vi "SDT_WriteFile.vi"(5 "ActiveModule":string[](array[string]), 7 "Data":T12, 8 "ErrorIn":errorcluster, 9 "SPCdata":T13={"base_adr"=52672, "init"=0, "cfd_limit_low"=-0.0, "cfd_limit_high"=5.019608, "cfd_zc_level"=-5.2913384, "cfd_holdoff"=5.0, "sync_zc_level"=-5.2913384, "sync_holdoff"=4.0, "sync_threshold"=-70.588234, "tac_range"=50.033573, "sync_freq_div"=1, "tac_gain"=1, "tac_offset"=5.098039, "tac_limit_low"=0.0, "tac_limit_high"=100.0, "adc_resolution"=12, "ext_latch_delay"=0, "collect_time"=1.0, "display_time"=1.0, "repeat_time"=10.0, "stop_on_time"=1, "stop_on_ovfl"=1, "dither_range"=128, "count_incr"=1, "mem_bank"=0, "dead_time_comp"=0, "scan_control"=0, "routing_mode"=0, "tac_enable_hold"=0.0, "pci_card_no"=-1, "mode"=5, "scan_size_x"=1, "scan_size_y"=1, "scan_rout_x"=1, "scan_rout_y"=1, "scan_flyback"=65537, "scan_borders"=0, "scan_polarity"=0, "pixel_clock"=1, "line_compression"=1, "trigger"=0, "pixel_time"=1e-07, "ext_pixclk_div"=1, "rate_count_time"=1.0, "macro_time_clk"=0, "add_select"=0, "test_eep"=1, "adc_zoom"=0, "img_size_x"=1, "img_size_y"=1, "img_rout_x"=1, "img_rout_y"=1, "xy_gain"=1, "master_clock"=0, "adc_sample_delay"=0, "detector_type"=1, "chan_enable"=4191231, "chan_slope"=0, "chan_spec_no"=34835, "tdc_control"=0, "tdc_offset1"=0.0, "tdc_offset2"=0.0, "tdc_offset3"=0.0, "tdc_offset4"=0.0, "tdc_offset5"=0.0, "tdc_offset6"=0.0, "cfd_th5_tdc"=0.0, "cfd_th6_tdc"=0.0, "cfd_zc5_tdc"=0.0, "cfd_zc6_tdc"=0.0, "future_reserve1"=0, "future_reserve2"=0, "future_reserve3"=0, "future_reserve4"=0} {"scan_flyback" format="%x"}, 10 "ImageSize":i32=256, 11 "SDT-FilePath":path=path "\\\\lab13\\C/Users/jannis/Desktop/ZeissFifo.sdt") -> (0 "ErrorOut":errorcluster)   [LabVIEW 2017]
doc: "This VI writes a SDT-file to disc. The SetUp and the MeasureInfo blocks are created and appended with the data blocks. \nThis VI is limited to writing a DecayMatrix from a FIFO-Image recording and optional an IntensityImage to file. For single mode recordings use the spcmdll VI \\Public\\Configure\\Memory Transfer\\SPC_save_data_to_sdtfile.vi.\nFor a description of the format for the Data input cluster to this VI see the usage in \\Example\\ImagingEventStream-SimpleFifoImage.vi. Leave either of the cluster input arrays empty to not save them to disc.\nFor a description of the *.sdt file format see: SPC_data_file_structure.h\n\ninfo@becker-hickl.com"
uses:
  SPC_Wrappers/SPC_Controls/bhfile_header.ctl
  SPC_Wrappers/SPC_Controls/SPCdata.ctl
  SPC_Wrappers/SPC_Controls/MeasureInfo.ctl
  SPC_Wrappers/SPC_Controls/MeasureInfo_PartB.ctl
  SPC_Wrappers/SPC_Controls/MeasStopInfo.ctl
  SPC_Wrappers/SPC_Controls/MeasFCSInfo.ctl
  SPC_Wrappers/SPC_Controls/MeasureInfo_PartE.ctl
  SPC_Wrappers/SPC_Controls/MeasHISTInfo.ctl
  SPC_Wrappers/SPC_Controls/HISTInfoExt.ctl
  SPC_Wrappers/SPC_Controls/MeasureInfo_PartI.ctl
  SPC_Wrappers/SPC_Controls/MeasureInfo_PartK.ctl
  SPC_Wrappers/SPC_Controls/MeasureInfo_PartM.ctl
  SPC_Wrappers/SPC_Controls/BHFileBlockHeader.ctl
  SPC_Wrappers/SPC_Controls/FileType.ctl
  SDT_CreateModTypeString.vi
  SDT_MeasureBlockToString.vi
panel:
  out "Info Block":string
  out "BHFileBlockHeaders":T1[](array[typedef])
  out "MeasureInfos":T2[](array[typedef]) {"MeasStopInfo"."flags" format="x%x"}
  out "BlockLengths":i32[](array[numeric])
  out "bhfile_header":T14 {"chksum" format="x%x"; "header_valid" format="x%x"}
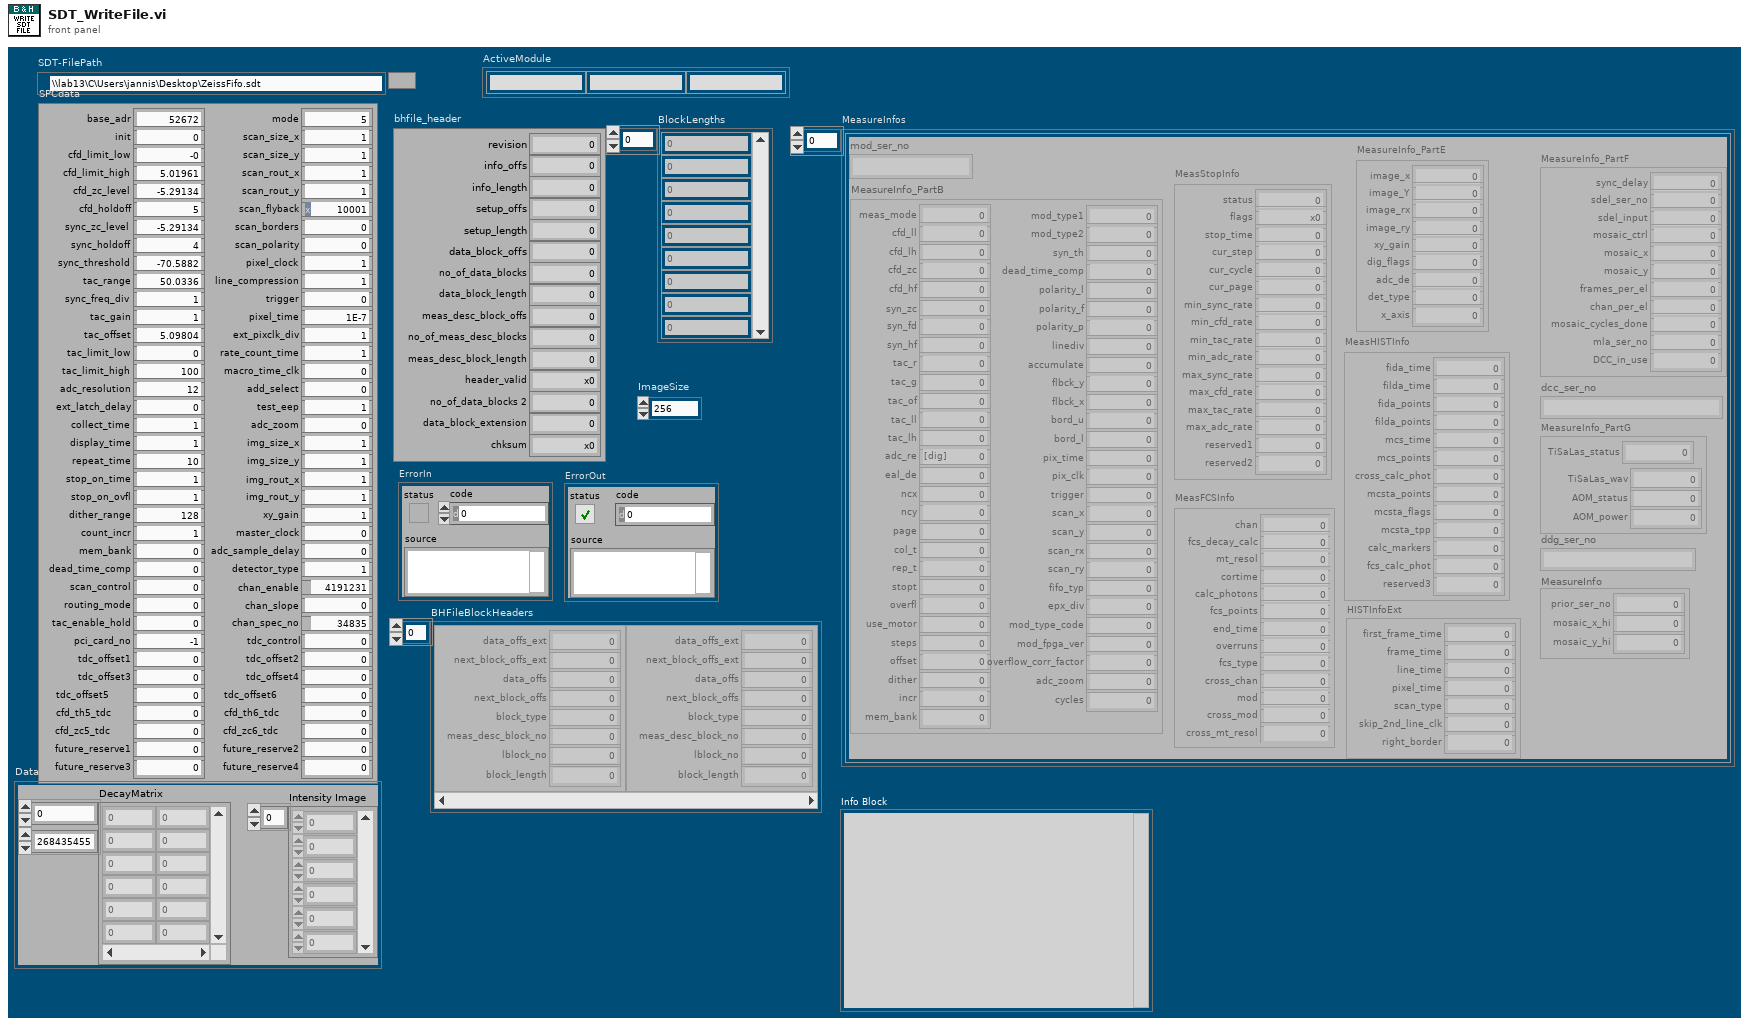
[diagram p1: front panel]
types:
  T1 = typedef "BHFileBlockHeader.ctl" = cluster{"data_offs_ext":u8, "next_block_offs_ext":u8, "data_offs":u32, "next_block_offs":u32, "block_type":u16, "meas_desc_block_no":i16, "lblock_no":u32, "block_length":u32}
  T2 = typedef "MeasureInfo.ctl" = cluster{"mod_ser_no":string, "MeasureInfo_PartB":T3, "MeasStopInfo":T4, "MeasFCSInfo":T5, "MeasureInfo_PartE":T6, "MeasHISTInfo":T7, "HISTInfoExt":T8, "MeasureInfo_PartF":T9, "dcc_ser_no":string, "MeasureInfo_PartG":T10, "ddg_ser_no":string, "MeasureInfo":T11}
  T3 = typedef "MeasureInfo_PartB.ctl" = cluster{"meas_mode":i16, "cfd_ll":sgl, "cfd_lh":sgl, "cfd_zc":sgl, "cfd_hf":sgl, "syn_zc":sgl, "syn_fd":i16, "syn_hf":sgl, "tac_r":sgl, "tac_g":i16, "tac_of":sgl, "tac_ll":sgl, "tac_lh":sgl, "adc_re":i16, "eal_de":i16, "ncx":i16, "ncy":i16, "page":u16, "col_t":sgl, "rep_t":sgl, "stopt":i16, "overfl":i8, "use_motor":i16, "steps":u16, "offset":sgl, "dither":i16, "incr":i16, "mem_bank":i16, "mod_type1":u64, "mod_type2":u64, "syn_th":sgl, "dead_time_comp":i16, "polarity_l":i16, "polarity_f":i16, "polarity_p":i16, "linediv":i16, "accumulate":i16, "flbck_y":i32, "flbck_x":i32, "bord_u":i32, "bord_l":i32, "pix_time":sgl, "pix_clk":i16, "trigger":i16, "scan_x":i32, "scan_y":i32, "scan_rx":i32, "scan_ry":i32, "fifo_typ":i16, "epx_div":i32, "mod_type_code":u16, "mod_fpga_ver":u16, "overflow_corr_factor":sgl, "adc_zoom":i32, "cycles":i32}
  T4 = typedef "MeasStopInfo.ctl" = cluster{"status":u16, "flags":u16, "stop_time":sgl, "cur_step":i32, "cur_cycle":i32, "cur_page":i32, "min_sync_rate":sgl, "min_cfd_rate":sgl, "min_tac_rate":sgl, "min_adc_rate":sgl, "max_sync_rate":sgl, "max_cfd_rate":sgl, "max_tac_rate":sgl, "max_adc_rate":sgl, "reserved1":i32, "reserved2":sgl}
  T5 = typedef "MeasFCSInfo.ctl" = cluster{"chan":u16, "fcs_decay_calc":u16, "mt_resol":u32, "cortime":sgl, "calc_photons":u32, "fcs_points":i32, "end_time":sgl, "overruns":u16, "fcs_type":u16, "cross_chan":u16, "mod":u16, "cross_mod":u16, "cross_mt_resol":u32}
  T6 = typedef "MeasureInfo_PartE.ctl" = cluster{"image_x":i32, "image_Y":i32, "image_rx":i32, "image_ry":i32, "xy_gain":i16, "dig_flags":i16, "adc_de":i16, "det_type":i16, "x_axis":i16}
  T7 = typedef "MeasHISTInfo.ctl" = cluster{"fida_time":sgl, "filda_time":sgl, "fida_points":i32, "filda_points":i32, "mcs_time":sgl, "mcs_points":i32, "cross_calc_phot":u32, "mcsta_points":u16, "mcsta_flags":u16, "mcsta_tpp":u32, "calc_markers":u32, "fcs_calc_phot":u32, "reserved3":u32}
  T8 = typedef "HISTInfoExt.ctl" = cluster{"first_frame_time":sgl, "frame_time":sgl, "line_time":sgl, "pixel_time":sgl, "scan_type":i16, "skip_2nd_line_clk":i16, "right_border":u32}
  T9 = typedef "MeasureInfo_PartI.ctl" = cluster{"sync_delay":sgl, "sdel_ser_no":u16, "sdel_input":i8, "mosaic_ctrl":i8, "mosaic_x":u8, "mosaic_y":u8, "frames_per_el":i16, "chan_per_el":i16, "mosaic_cycles_done":i32, "mla_ser_no":u16, "DCC_in_use":u8}
  T10 = typedef "MeasureInfo_PartK.ctl" = cluster{"TiSaLas_status":u16, "TiSaLas_wav":u16, "AOM_status":u8, "AOM_power":u8}
  T11 = typedef "MeasureInfo_PartM.ctl" = cluster{"prior_ser_no":i32, "mosaic_x_hi":u8, "mosaic_y_hi":u8}
  T12 = cluster{"DecayMatrix":u16[][], "Intensity Image":u32[]}
  T13 = typedef "SPCdata.ctl" = cluster{"base_adr":u16, "init":i16, "cfd_limit_low":sgl, "cfd_limit_high":sgl, "cfd_zc_level":sgl, "cfd_holdoff":sgl, "sync_zc_level":sgl, "sync_holdoff":sgl, "sync_threshold":sgl, "tac_range":sgl, "sync_freq_div":i16, "tac_gain":i16, "tac_offset":sgl, "tac_limit_low":sgl, "tac_limit_high":sgl, "adc_resolution":i16, "ext_latch_delay":i16, "collect_time":sgl, "display_time":sgl, "repeat_time":sgl, "stop_on_time":i16, "stop_on_ovfl":i16, "dither_range":i16, "count_incr":i16, "mem_bank":i16, "dead_time_comp":i16, "scan_control":u16, "routing_mode":u16, "tac_enable_hold":sgl, "pci_card_no":i16, "mode":u16, "scan_size_x":u32, "scan_size_y":u32, "scan_rout_x":u32, "scan_rout_y":u32, "scan_flyback":u32, "scan_borders":u32, "scan_polarity":u16, "pixel_clock":u16, "line_compression":u16, "trigger":u16, "pixel_time":sgl, "ext_pixclk_div":u32, "rate_count_time":sgl, "macro_time_clk":i16, "add_select":i16, "test_eep":i16, "adc_zoom":i16, "img_size_x":u32, "img_size_y":u32, "img_rout_x":u32, "img_rout_y":u32, "xy_gain":i16, "master_clock":i16, "adc_sample_delay":i16, "detector_type":i16, "chan_enable":u32, "chan_slope":u32, "chan_spec_no":u32, "tdc_control":u32, "tdc_offset1":sgl, "tdc_offset2":sgl, "tdc_offset3":sgl, "tdc_offset4":sgl, "tdc_offset5":sgl, "tdc_offset6":sgl, "cfd_th5_tdc":sgl, "cfd_th6_tdc":sgl, "cfd_zc5_tdc":sgl, "cfd_zc6_tdc":sgl, "future_reserve1":u64, "future_reserve2":u64, "future_reserve3":u64, "future_reserve4":u64}
  T14 = typedef "bhfile_header.ctl" = cluster{"revision":i16, "info_offs":i32, "info_length":i16, "setup_offs":i32, "setup_length":u16, "data_block_offs":i32, "no_of_data_blocks":i16, "data_block_length":u32, "meas_desc_block_offs":i32, "no_of_meas_desc_blocks":i16, "meas_desc_block_length":i16, "header_valid":u16, "no_of_data_blocks 2":u32, "data_block_extension":u16, "chksum":u16}
  T15 = typedef "FileType.ctl" = u16
  T16 = enum16{"open", "replace", "create", "open or create", "replace or create", "replace or create with confirmation"}
  T17 = enum16{"big-endian, network order", "native, host order", "little-endian"}
  T18 = typedef "BHModuleType.ctl" = i16
  T19 = typedef "ModuleType.ctl" = i16
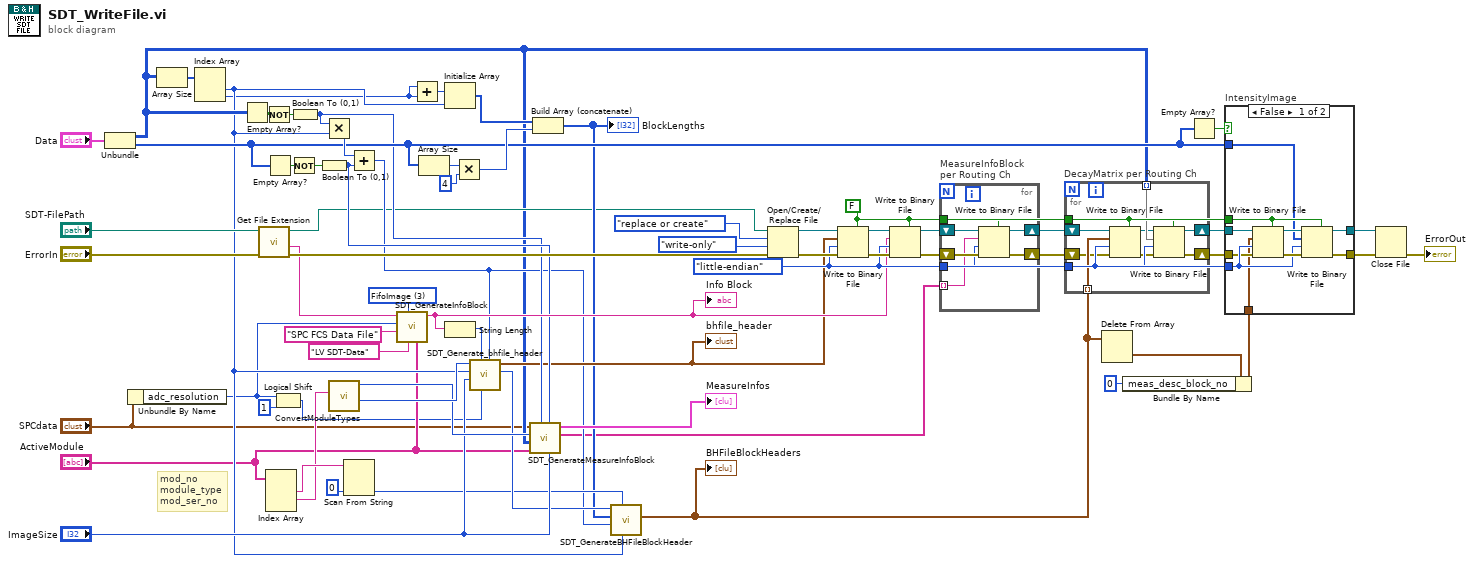
[diagram p0: block diagram]
diagram:
  w6 = T15 3 items=["non-Fifo"=1, "Fifo"=2, "FifoImage"=3] ("FileType")
  w57 = FALSE ("prepend array or string size? (T)")
  w56 = T17."little-endian" ("byte order (0:big-endian, network order)")
  # "mod_no\nmodule_type\nmod_ser_no"
  n1 = Unbundle("Data") -> ("DecayMatrix"=w9:u16[][], "Intensity Image"=w30:u32[])
  n2 = Unbundle By Name("SPCdata") -> ("adc_resolution"=w3:i16)
  n3 = Array Size(array=w9) -> (size(s)=w39:i32[])
  n4 = Index Array(array=w39) -> (element #1=w8:i32, element #2=w7:i32)  [unwired: 2 in]
  n5 = Empty Array?(array=w9) -> (empty?=w49:bool)
  n6 = call <vilib>:"Get File Extension.vi"("error in (no error)"="ErrorIn", "file"="SDT-FilePath") -> ("error out"=w63:errorcluster, "filename without extension"=w29:string, "dup file"=w11:path)  [unwired: 5 in, 2 out]
  n7 = Not(x=w49) -> (.not. x?=w47:bool)
  n8 = Empty Array?(array=w30) -> (empty?=w48:bool)
  n9 = Index Array(array="ActiveModule") -> (element #1=w45:string, element #2=w41:string)  [unwired: 3 in, 1 out]
  n10 = Logical Shift(y=w3, x=u32 1) -> (x << y=w1:u32)
  n11 = Not(x=w48) -> (.not. x?=w46:bool)
  n12 = Boolean To (0,1)(Boolean=w47) -> (0, 1=w19:i16)
  n13 = Boolean To (0,1)(Boolean=w46) -> (0, 1=w23:i16)
  n14 = Multiply(x=w19, y=w8) -> (x*y=w36:i32)
  n15 = call "ConvertModuleTypes.vi"("ModuleTypeStringIn"=w41) -> ("BHModuleType"=w24:T18, "Module TypeOut"=w22:T19)  [unwired: 8 in, 1 out]
  n16 = Scan From String(input string=w45, default 1=u32 0 ("meas_desc_block_no")) -> (output 1=w15:u32)  [unwired: 3 in, 3 out]
  n17 = Add(x=w36, y=w23) -> (x+y=w13:i32)
  n18 = call "SDT_GenerateInfoBlock.vi"("ActiveModule"="ActiveModule", "Contents"="LV SDT-Data", "FileType"=w6, "FileID"="SPC FCS Data File", "adc_re[exp]"=w3, "FilenameNoExtension"=w29) -> ("Info Block"=w26:string)  [unwired: 5 in]
  "Info Block" <- w26
  n19 = Add(x=w7, y=w7) -> (x+y=w38:i32)
  n20 = Array Size(array=w30) -> (size(s)=w51:i32)
  n21 = Initialize Array(w38, w8) -> (w37:i32[])
  n22 = String Length(string=w26) -> (length=w25:i32)
  n23 = Multiply(x=w51, y=4) -> (x*y=w43:i32)
  n24 = call "SDT_Generate_bhfile_header.vi"("no_of_data_blocks"=w13, "adc_re[dig]"=w1, "info_length"=w25, "ImageSize"="ImageSize", "NoOfRoutingChannel"=w8, "BHModuleType"=w24) -> ("data_block_offs"=w16:i32, "bhfile_header"=w18:T14)  [unwired: 4 in]
  "bhfile_header" <- w18
  n25 = call "SDT_GenerateMeasureInfoBlock.vi"("ImageSize"="ImageSize", "HasIntensityImage"=w23, "HasFifoImage"=w19, "ActiveModule"="ActiveModule", "DecayMatrix"=w9, "Module Type"=w22, "SPCdata"="SPCdata") -> ("MeasureInfoStrings"=w10:string[], "MeasureInfos"=→"MeasureInfos":T2[])  [unwired: 3 in]
  n26 = Build Array (concatenate)(w37, w43) -> (w14:i32[])
  "BlockLengths" <- w14
  n27 = call "SDT_GenerateBHFileBlockHeader.vi"("NoOfRoutingChannels"=w8, "ModuleNo"=w15, "NoOfDataBlocks"=w13, "BlockLengths"=w14, "data_block_offs"=w16) -> ("BHFileBlockHeaders"=w17:T1[])  [unwired: 5 in, 1 out]
  "BHFileBlockHeaders" <- w17
  n28 = Open/Create/Replace File(file path (use dialog)=w11, error in=w63, operation (0:open)=T16."replace or create", access (0:read/write)=enum16{"read/write", "read-only", "write-only"}."write-only") -> (refnum out=w66:refnum<file>, error out=w62:errorcluster)  [unwired: 2 in, 1 out]
  n29 = Write to Binary File(file (use dialog)=w66, data=w18, error in=w62, 5:w57, 9:w56) -> (refnum out=w65:refnum<file>, error out=w61:errorcluster)  [unwired: 1 in, 1 out]
  n30 = Write to Binary File(file (use dialog)=w65, data=w26, error in=w61, 5:w57, 9:w56) -> (refnum out=w64:refnum<file>, error out=w60:errorcluster)  [unwired: 1 in, 1 out]
  n31 = for "MeasureInfoBlock\nper Routing Ch" {
    tunnel: w57 -> [w73]
    tunnel: w56 -> [w72]
    shift-right: [w71] -> w35
    shift-left: w64 -> [w75]
    shift-right: [w70] -> w34
    shift-left: w60 -> [w74]
    tunnel: w10 -> [w69] mode=indexing
    n32 = Write to Binary File(file (use dialog)=w75, data=w69, error in=w74, 5:w73, 9:w72) -> (refnum out=w71:refnum<file>, error out=w70:errorcluster)  [unwired: 1 in, 1 out]
  }
  n33 = for "DecayMatrix per Routing Ch" {
    tunnel: w57 -> [w85]
    tunnel: w56 -> [w84]
    tunnel: w17 -> [w81] mode=indexing
    tunnel: w9 -> [w80] mode=indexing
    shift-right: [w82] -> w54
    shift-left: w35 -> [w79]
    shift-right: [w83] -> w55
    shift-left: w34 -> [w78]
    n34 = Write to Binary File(file (use dialog)=w79, data=w81, error in=w78, 5:w85, 9:w84) -> (refnum out=w77:refnum<file>, error out=w76:errorcluster)  [unwired: 1 in, 1 out]
    n35 = Write to Binary File(file (use dialog)=w77, data=w80, error in=w76, 5:w85, 9:w84) -> (refnum out=w82:refnum<file>, error out=w83:errorcluster)  [unwired: 1 in, 1 out]
  }
  n36 = Delete From Array(array=w17) -> (deleted portion=w40:T1)  [unwired: 2 in, 1 out]
  n37 = Bundle By Name(cluster=w40, "meas_desc_block_no"=i16 0) -> (w33:T1)
  n38 = Empty Array?(array=w30) -> (empty?=w31:bool)
  n39 = case "IntensityImage" shown="False" w31 {
    tunnel: w57 -> [w93 _]
    tunnel: w56 -> [w92 _]
    tunnel: w55 -> [w91 w96]
    tunnel: w54 -> [w90 w97]
    tunnel: [w89 w96] -> w53
    tunnel: [w88 w97] -> w52
    tunnel: w30 -> [w87 _]
    tunnel: w33 -> [w86 _]
    frame False {
      n40 = Write to Binary File(file (use dialog)=w90, data=w86, error in=w91, 5:w93, 9:w92) -> (refnum out=w94:refnum<file>, error out=w95:errorcluster)  [unwired: 1 in, 1 out]
      n41 = Write to Binary File(file (use dialog)=w94, data=w87, error in=w95, 5:w93, 9:w92) -> (refnum out=w88:refnum<file>, error out=w89:errorcluster)  [unwired: 1 in, 1 out]
    }
    frame True {
    }
  }
  n42 = Close File(refnum=w52, error in=w53) -> (error out=→"ErrorOut":errorcluster)  [unwired: 1 out]
